vi "Measurement UI.vi"() -> ()   [LabVIEW 2021, in "Stepped Frequency Sweep_Class D Amplifier_UI.lvlib"]
uses:
  Stepped Frequency Sweep_Class D Amplifier_UI.lvlib
  shared/controls/sweep profile.ctl
  shared/controls/units - snr.ctl
  shared/controls/units - ratio.ctl
  Y axis data selection.ctl
  shared/controls/digital output level units.ctl
  shared/ui/controls/view.ctl
  UI State.ctl
  <vilib>/Utility/miscctls.llb/LVBoundsTypeDef.ctl
  <vilib>/Utility/miscctls.llb/LVPoint32TypeDef.ctl
  shared/ui/UI Helpers.lvlib
  shared/controls/audio controls.lvlib
panel:
  in  "view legend":T1
  out "Sweep graph":cluster{"frequency (Hz)":dbl[], "THD+N":dbl[]}[](graph)
  out "Time domain graph":waveform(dbl)(graph)
  out "Frequency domain graph":T2(graph)
  out "amplitude (Vrms)":dbl[](array[numeric])
  out "output power (W)":dbl[](array[numeric])
  out "SFDR (dBc)":dbl[](array[numeric])
  out "gain":dbl[](array[numeric])
  out "dynamic range (dB)":dbl[](array[numeric])
  out "THD":dbl[](array[numeric])
  out "THD+N":dbl[](array[numeric])
  out "SNR":dbl[](array[numeric])
  out "amplitude (dBFS)":dbl[](array[numeric])
  out "frequency (Hz)":dbl[](array[numeric])
  in  "Configuration tab":T3(tab)
  in  "enable dither":bool caption="Enable dither"
  in  "master clock channel list":string caption="Master Clock Channel"
  in  "digital channel list":string caption="Digital Audio Channel"
  in  "logic level":enum32{"3.3 V", "1.8 V", "1.2 V"}(ring) caption="Logic level"
  in  "master clock rate":dbl=12288000.0 caption="Master clock rate" format="%#_6pHz"
  out "Bit clock rate":dbl=3072000.0 format="%#_6pHz"
  in  "number of channels":u32=2 caption="Number of channels"
  in  "TDM":bool
  in  "RJ":bool
  in  "LJ":bool
  in  "I2S":bool
  in  "bit clock edge sync":enum32{"Rising", "Falling"}(ring)=enum."Falling" caption="Bit clock edge sync"
  in  "frame clock rate":dbl=48000.0 caption="Frame clock rate" format="%#_6pHz"
  in  "data justification":enum32{"Left Justified", "Right Justified"}(ring) caption="Data justification"
  in  "endianness":enum32{"MSB First", "LSB First"}(ring) caption="Endianness"
  in  "bit depth":u32=24 caption="Bit depth"
  in  "channel length":u32=32 caption="Channel length"
  in  "frame sync edge for channel 0":enum32{"Rising", "Falling"}(ring)=enum."Falling" caption="Frame sync edge for Channel 0"
  in  "output level":dbl=-1.0 caption="Output level" format="%#_3f"
  in  "output level units":T4
  in  "min settling cycles":u32 caption="Minimum settling cycles"
  in  "min settling time (s)":dbl=0.1 caption="Minimum settling time" format="%#_6ps"
  in  "sweep profile":T5=enum."Logarithmic" caption="Profile"
  in  "number of steps":u32=20000 caption="Number of steps"
  in  "sweep start frequency (Hz)":dbl=20.0 caption="Sweep start" format="%#_6pHz"
  in  "sweep stop frequency (Hz)":dbl=20000.0 caption="Sweep stop" format="%#_6pHz"
  in  "min measurement cycles":u32 caption="Minimum measurement cycles"
  in  "Acquisition channel":tag
  in  "acq sampling rate":dbl=51200.0 caption="Sample rate" format="%#.6pHz"
  in  "min measurement time (s)":dbl=0.1 caption="Minimum measurement time" format="%#_6ps"
  in  "lowpass filter":T6(ring) caption="Lowpass filter"
  in  "highpass filter":enum32{"DC", "AC"}(ring) caption="Highpass filter"
  in  "band start":dbl=20.0 caption="Band start" format="%#_6pHz"
  in  "band stop":dbl=20000.0 caption="Band stop" format="%#_6pHz"
  in  "weighting filter":T7(ring)=enum."A-weighting" caption="Weighting filter"
  in  "load impedance":dbl=4.0 caption="Load impedance" format="%#_6p Ohms"
  in  "output range (pk-pk)":dbl=15.0 caption="Output range" format="%.3p Vpk-pk"
  in  "gain units":T8 caption="Gain"
  in  "THD units":T8 caption="THD"
  in  "THD+N units":T8 caption="THD+N"
  in  "SNR units":T9 caption="SNR"
  in  "x-axis mapping":enum32{"linear", "logarithmic"}(ring) caption="X-axis mapping"
  in  "y-axis mapping":enum32{"linear", "logarithmic"}(ring) caption="Y-axis mapping"
  in  "y-axis data":T10 caption="Y-axis"
  in  "channel 0 offset":u32=1
  out "fft - data":dbl[](array[numeric])
  out "fft - df":dbl
  out "fft - f0":dbl
  out "wfm - data":dbl[](array[numeric])
  out "wfm - dt":dbl
  out "wfm - t0":dbl
  out "channel name":string
  in  "acq channel":string="PXI1Slot4/ai0"
  in  "signal phase":dbl caption="phase"
  # "hidden controls - used to sync with MeasLink"
  # "hidden indicators"
  # "Protocols"
  # "Audio Protocol"
  # "Clock Settings"
  # "Signal Level"
  # "Harware Resource"
  # "Sweep"
  # "Filters"
  # "Output"
  # "Acquisition"
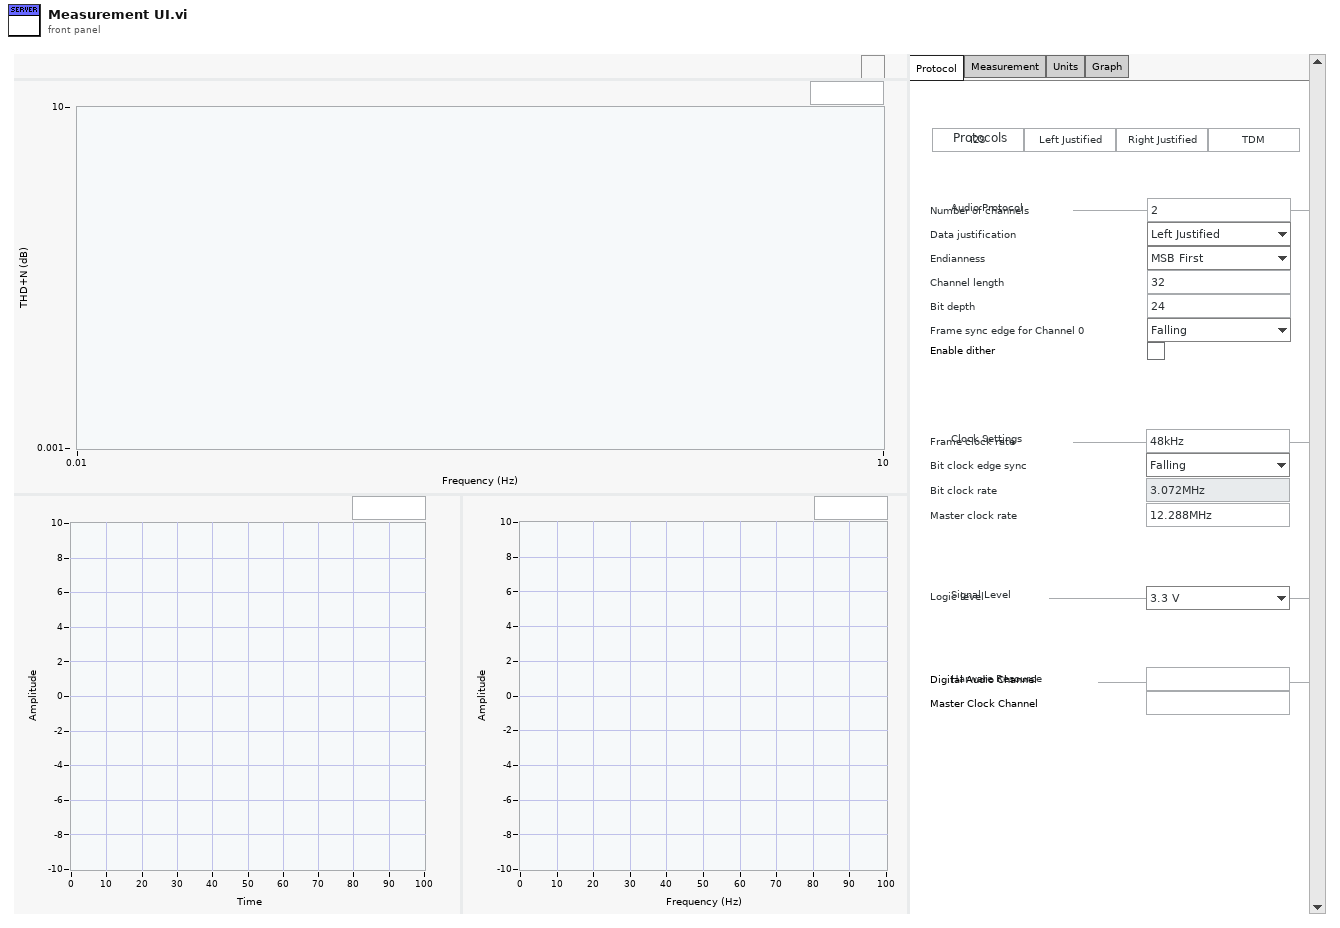
[diagram p1: front panel]
types:
  T1 = typedef "UI Helpers.lvlib/view.ctl" = bool
  T2 = cluster{"fft - f0":dbl, "fft - df":dbl, "fft - data":dbl[]}
  T3 = enum32{"Protocol", "Measurement", "Units", "Graph"}
  T4 = typedef "audio controls.lvlib/digital output level units.ctl" = enum32{"% FS", "dBFS"}
  T5 = typedef "audio controls.lvlib/sweep profile.ctl" = enum32{"Linear", "Logarithmic"}
  T6 = enum32{"No filter", "AES17 20kHz", "AES17 40kHz"}
  T7 = enum32{"Linear", "A-weighting", "B-weighting", "C-weighting"}
  T8 = typedef "audio controls.lvlib/units - ratio.ctl" = enum32{"dB", "%", "x/y"}
  T9 = typedef "audio controls.lvlib/units - snr.ctl" = enum32{"dB", "x/y"}
  T10 = typedef "Stepped Frequency Sweep_Class D Amplifier_UI.lvlib/Y axis data selection.ctl" = enum32{"THD+N", "THD", "Dynamic Range (dB)", "SFDR (dBc)", "SNR", "Gain", "Amplitude (dBFS)", "Amplitude (Vrms)", "Output Power (W)"}
  T11 = typedef "Stepped Frequency Sweep_Class D Amplifier_UI.lvlib/UI State.ctl" = cluster{"Graph Size":T12, "Legend Visible":bool, "Mouse Coords":T13}
  T12 = typedef "LVBoundsTypeDef.ctl" = cluster{"Width":u32, "Height":u32}
  T13 = typedef "LVPoint32TypeDef.ctl" = cluster{"Horizontal":i32, "Vertical":i32}
  T14 = cluster{"frequency (Hz)":dbl[], "amplitude (dBFS)":dbl[]}
  T15 = cluster{"frequency (Hz)":dbl[], "amplitude (Vrms)":dbl[]}
  T16 = cluster{"frequency (Hz)":dbl[], "output power (W)":dbl[]}
  T17 = cluster{"frequency (Hz)":dbl[], "dynamic range (dB)":dbl[]}
  T18 = cluster{"frequency (Hz)":dbl[], "SFDR (dBc)":dbl[]}
  T19 = cluster{"frequency (Hz)":dbl[], "SFDR (dBc)":dbl[]}[]
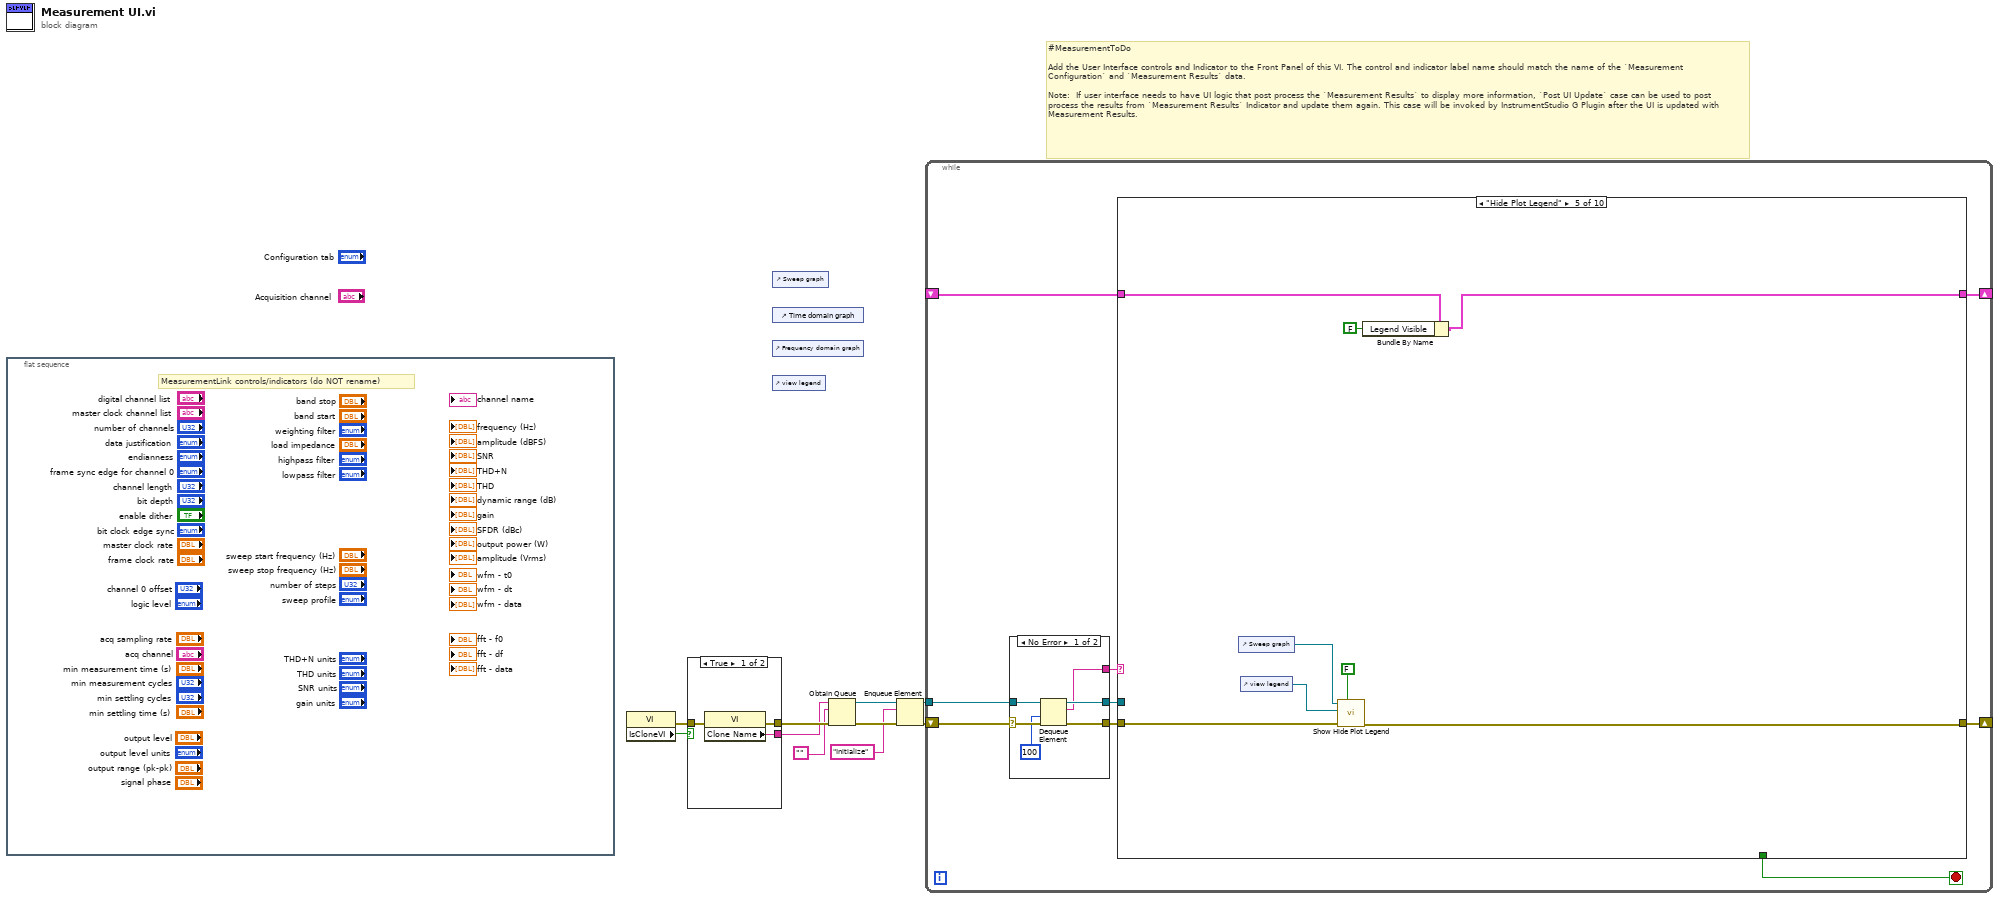
[diagram p0: block diagram]
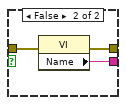
[diagram p2: hidden frame]
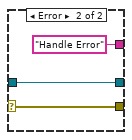
[diagram p3: hidden frame]
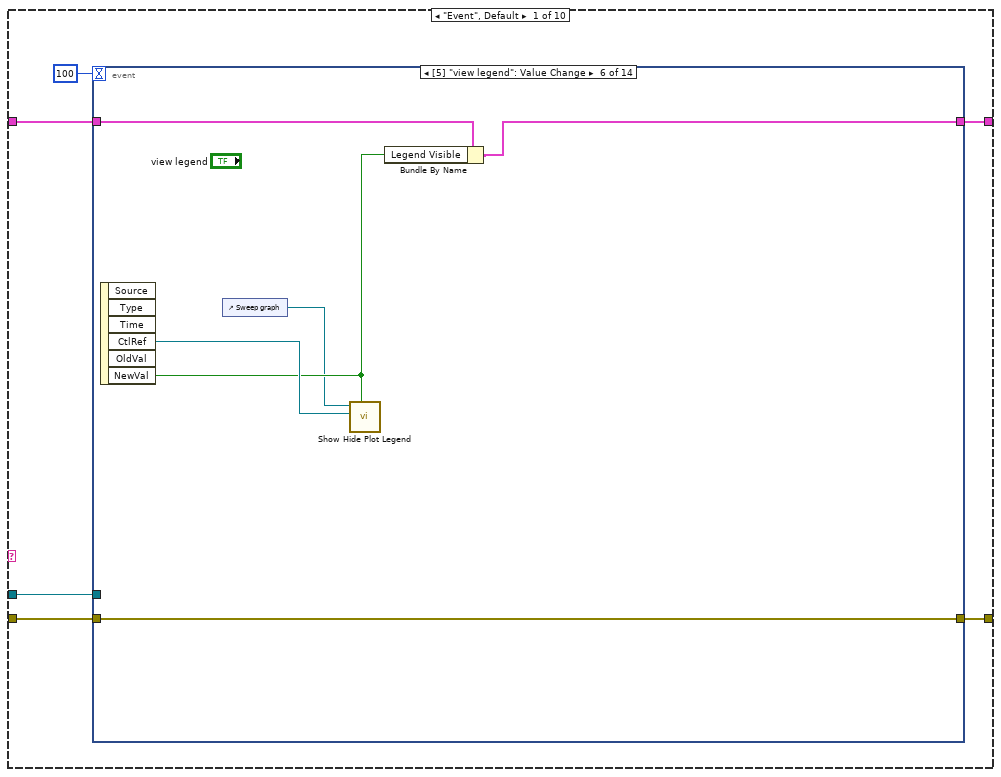
[diagram p4: hidden frame]
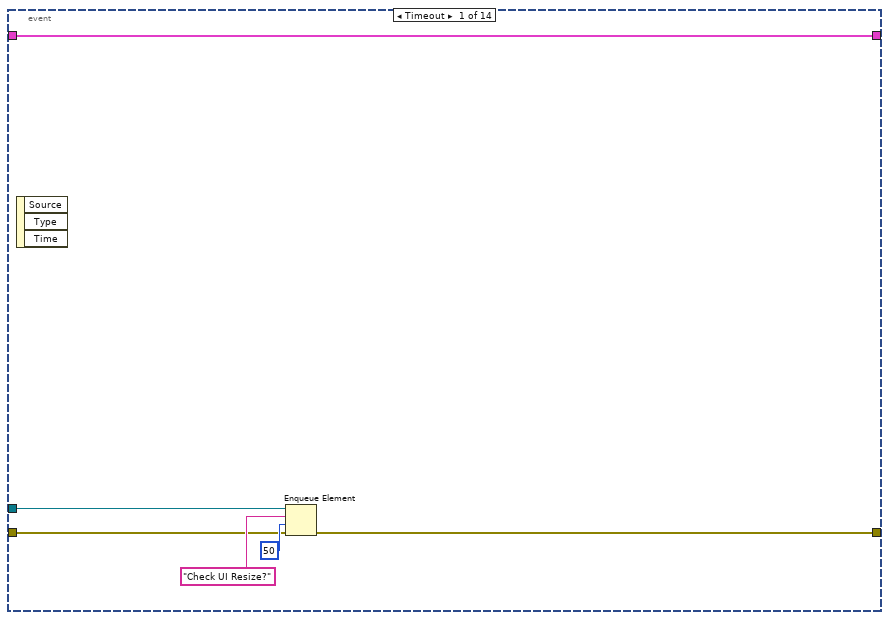
[diagram p5: hidden frame]
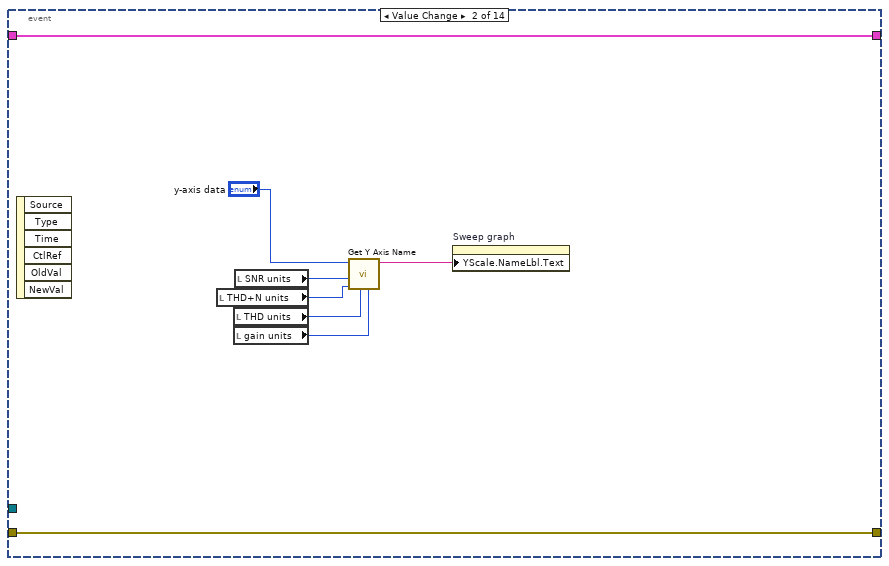
[diagram p6: hidden frame]
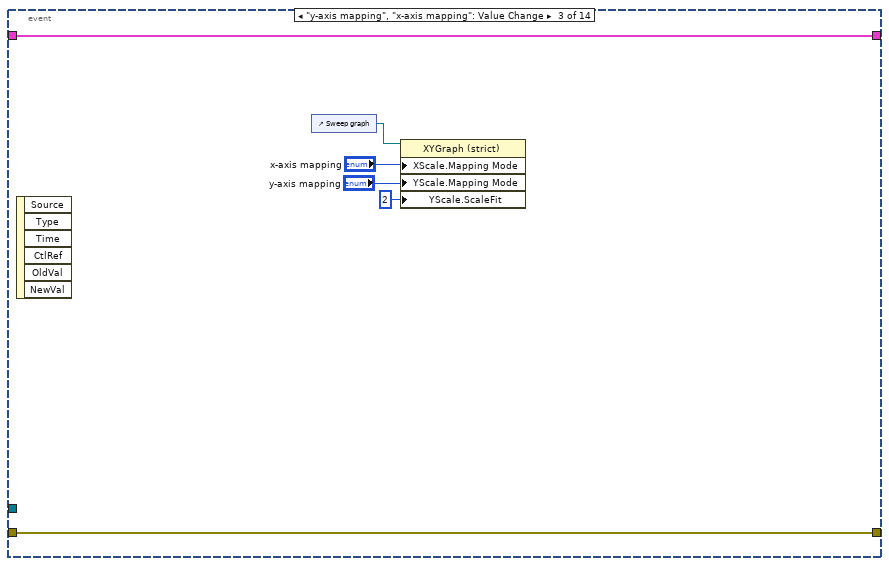
[diagram p7: hidden frame]
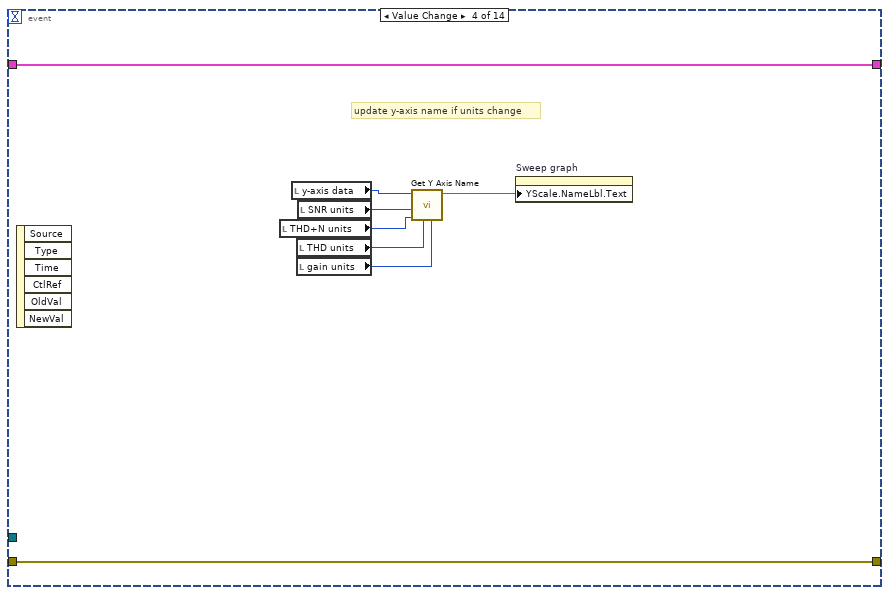
[diagram p8: hidden frame]
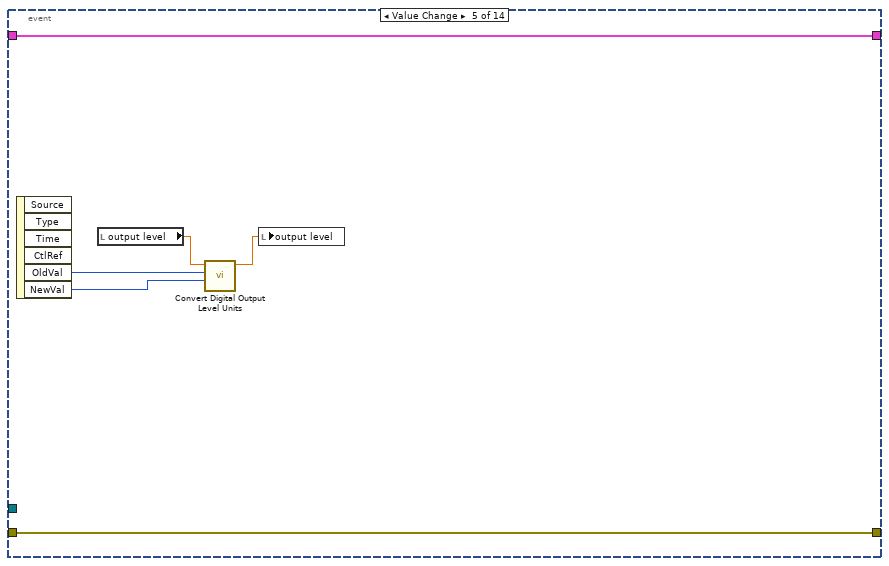
[diagram p9: hidden frame]
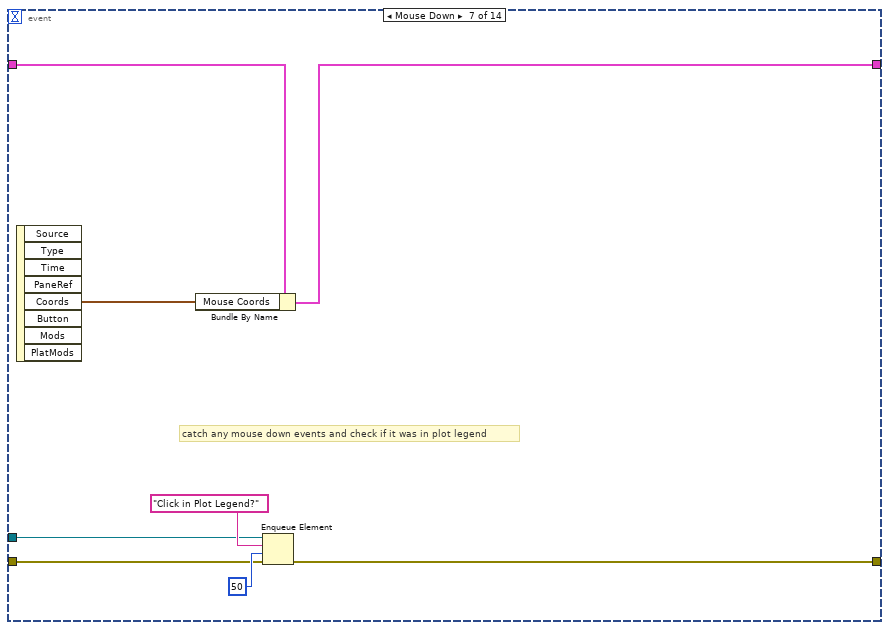
[diagram p10: hidden frame]
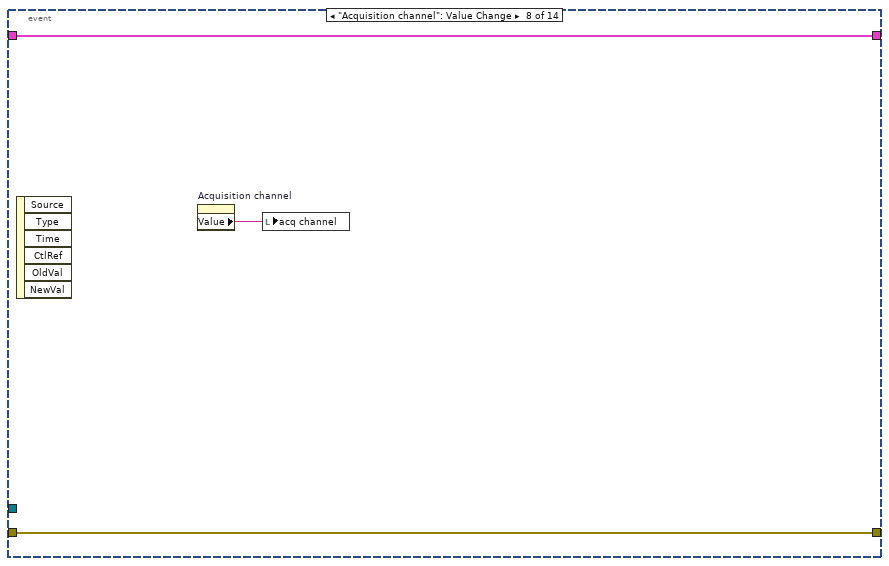
[diagram p11: hidden frame]
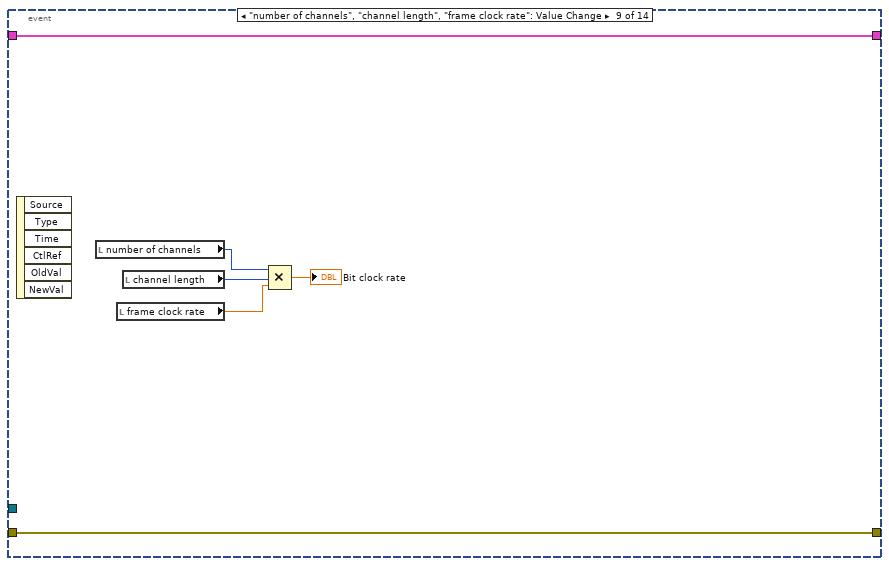
[diagram p12: hidden frame]
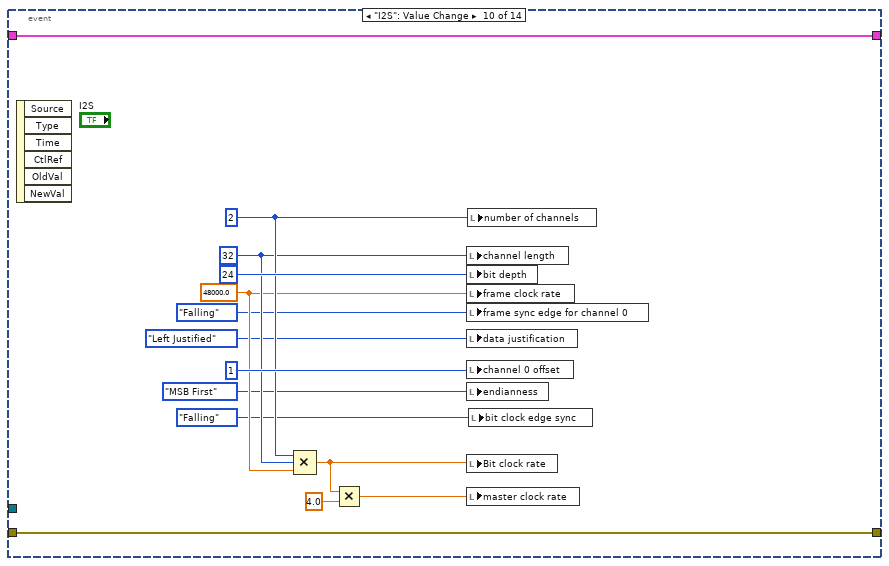
[diagram p13: hidden frame]
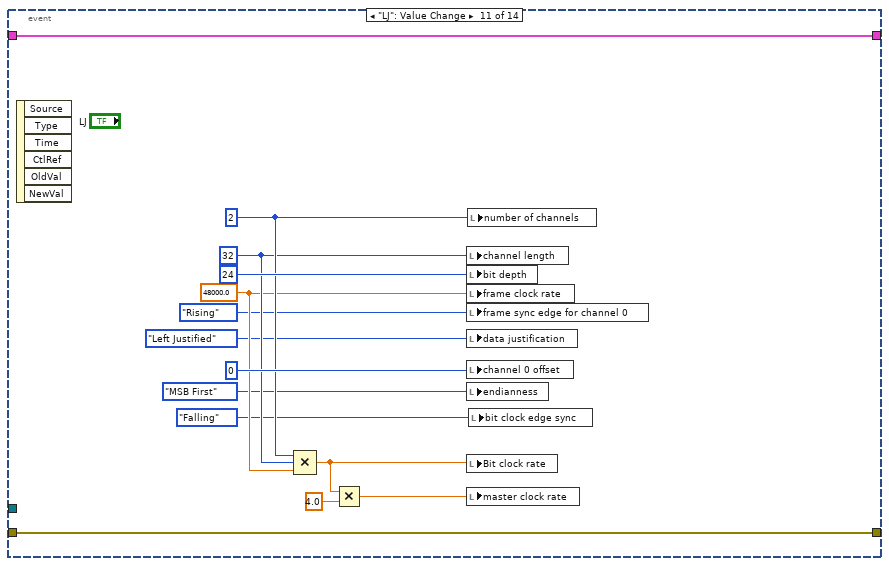
[diagram p14: hidden frame]
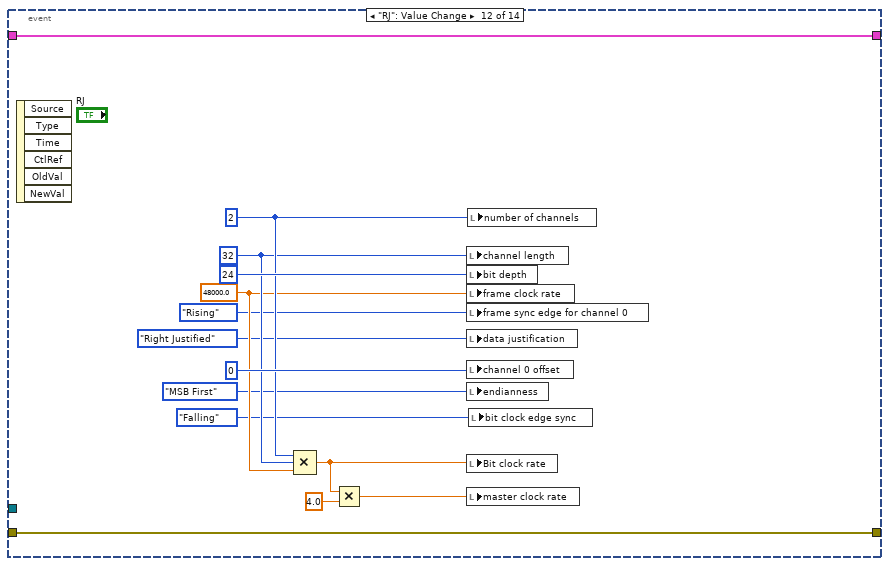
[diagram p15: hidden frame]
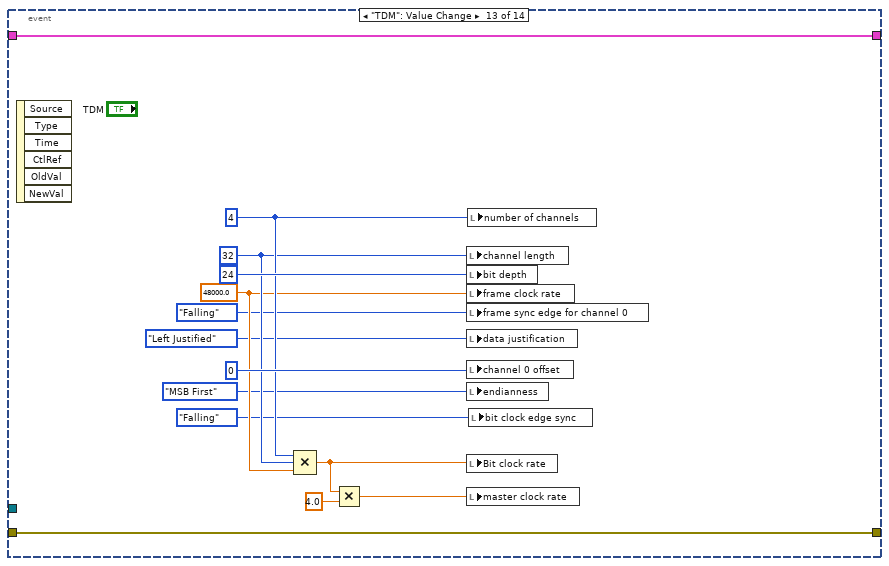
[diagram p16: hidden frame]
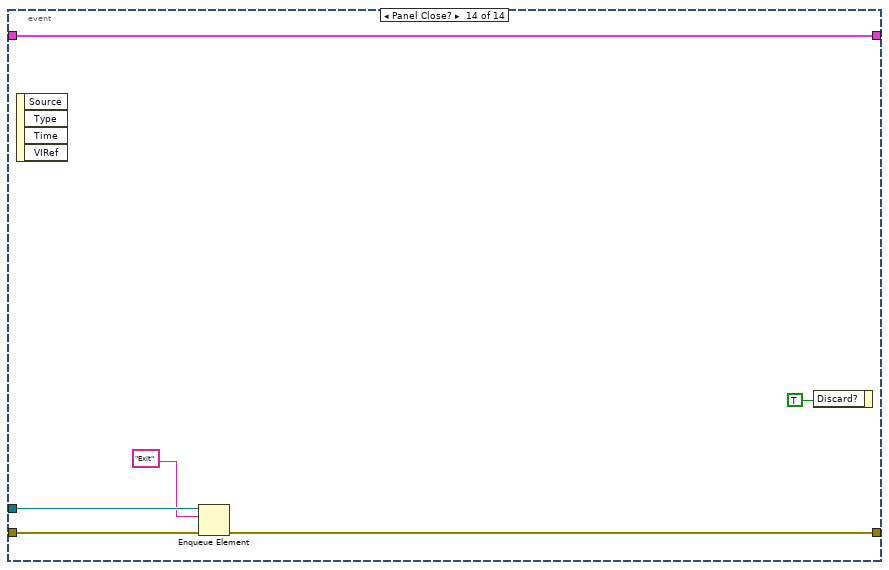
[diagram p17: hidden frame]
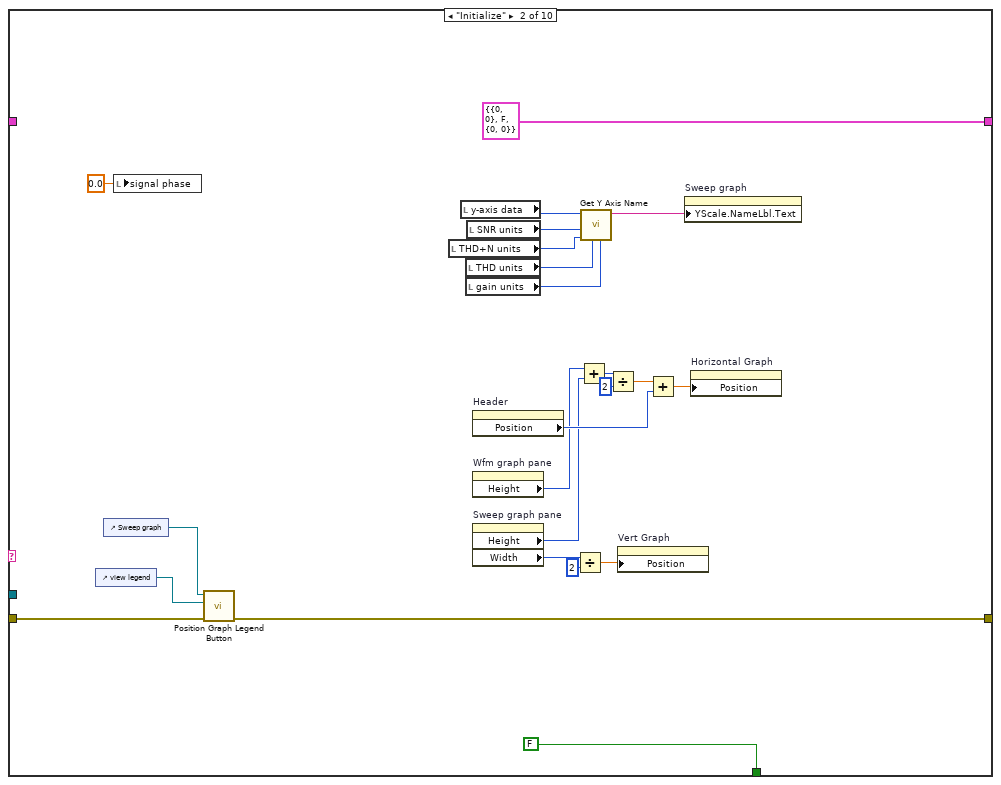
[diagram p18: hidden frame]
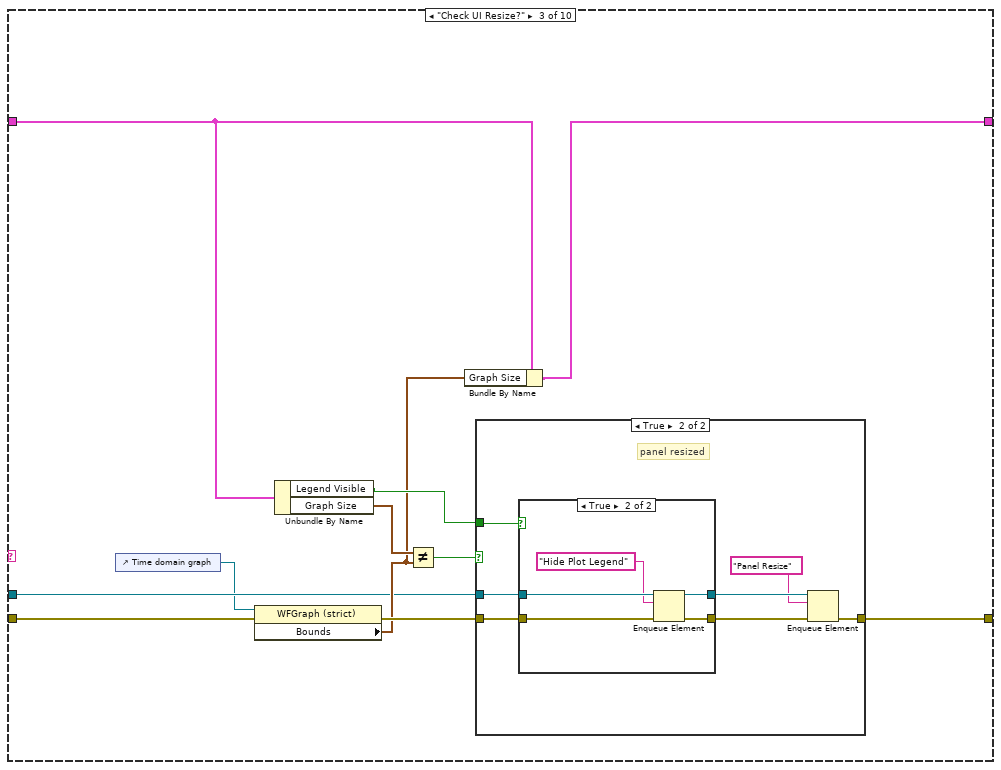
[diagram p19: hidden frame]
diagram:
  # "#MeasurementToDo  \n\nAdd the User Interface controls and Indicator to the Front Panel of this VI. The control and indicator label name should match the name of the `Measurement Configuration` and `Measurement Results` data.\n\nNote:  If user interface needs to have UI logic that post process the `Measurement Results` to display more information, `Post UI Update` case can be used to post process the results from `Measurement Results` Indicator and update them again. This case will be invoked by InstrumentStudio G Plugin after the UI is updated with Measurement Results."
  n1 = flat-sequence {
    frame #0 {
      # "MeasurementLink controls/indicators (do NOT rename)"
    }
  }
  n2 = property class="VI"() -> (error out=w1:errorcluster, "IsCloneVI"=w2:bool)  [unwired: 2 in, 1 out]
  n3 = case shown="True" w2 {
    tunnel: [w13 w16] -> w10
    tunnel: [w12 w15] -> w9
    tunnel: w1 -> [w11 w14]
    frame True {
      n4 = property class="VI"(error in=w11) -> (error out=w13:errorcluster, "Clone Name"=w12:string)  [unwired: 1 in, 1 out]
    }
    frame False {
      n5 = property class="VI"(error in=w14) -> (error out=w16:errorcluster, "Name"=w15:string)  [unwired: 1 in, 1 out]
    }
  }
  n6 = control-ref of="Sweep graph"() -> ()  [unwired: 1 out]
  n7 = control-ref of="Time domain graph"() -> ()  [unwired: 1 out]
  n8 = control-ref of="Frequency domain graph"() -> ()  [unwired: 1 out]
  n9 = control-ref of="view legend"() -> ()  [unwired: 1 out]
  n10 = Obtain Queue(name (unnamed)=w9, element data type="", error in (no error)=w10) -> (queue out=w6:refnum<queue>, error out=w8:errorcluster)  [unwired: 2 in, 1 out]
  n11 = Enqueue Element(queue=w6, element="Initialize", error in (no error)=w8) -> (queue out=w5:refnum<queue>, error out=w7:errorcluster)  [unwired: 1 in, 1 out]
  n12 = while {
    shift-right: [w20] -> _
    shift-left: w7 -> [w25]
    tunnel: w5 -> [w23]
    shift-right: [w18] -> _
    shift-left: _ -> [w17]
    stop <- w19 stop-if-true
    n13 = case shown="No Error" w25 {
      selector: w25 -> [w31 w34]
      tunnel: [w30 w34] -> w24
      tunnel: w23 -> [w29 w33]
      tunnel: [w28 w33] -> w22
      tunnel: [w27 "Handle Error"] -> w21
      frame No Error {
        n14 = Dequeue Element(queue=w29, timeout in ms (-1)=100, error in (no error)=w31) -> (queue out=w28:refnum<queue>, element=w27:string, error out=w30:errorcluster)  [unwired: 1 out]
      }
      frame Error {
      }
    }
    n15 = case shown="\"Hide Plot Legend\"" w21 {
      tunnel: w24 -> [w39 w174 w187 w211 w231 w239 w244 w277 w295 w297]
      tunnel: w22 -> [w37 _ w188 w212 _ _ w243 _ w293 _]
      tunnel: [w40 w173 w186 w210 w230 w238 w242 w277 w290 w297] -> w20
      tunnel: [_ FALSE _ _ _ _ _ _ TRUE _] -> w19
      tunnel: [w35 T11 {"Graph Size"={"Width"=0, "Height"=0}, "Legend Visible"=FALSE, "Mouse Coords"={"Horizontal"=0, "Vertical"=0}} ("UI State") w183 w209 w233 w240 w241 w276 w288 w296] -> w18
      tunnel: w17 -> [w36 _ w184 w209 w234 w240 w241 w276 w288 w296]
      frame "Event", Default {
        n16 = event shown="[5] \"view legend\": Value Change" {
          selector: _ -> [_ _ _ _ _ _ _ _ _ _ _ _ _ _]
          dyn-events: _ -> [_ _ _ _ _ _ _ _ _ _ _ _ _ _]
          timeout: 100 -> [_ _ _ _ _ _ _ _ _ _ _ _ _ _]
          tunnel: [w43 w47 w55 w61 w69 w80 w84 w89 w92 w98 w112 w126 w140 w157] -> w40
          tunnel: w39 -> [w44 w47 w55 w61 w69 w80 w86 w89 w92 w98 w112 w126 w140 w158]
          tunnel: w37 -> [w42 _ _ _ _ _ w85 _ _ _ _ _ _ w156]
          tunnel: w36 -> [w41 w48 w56 w62 w70 w77 w82 w90 w93 w99 w113 w127 w141 w154]
          tunnel: [w41 w48 w56 w62 w70 w76 w81 w90 w93 w99 w113 w127 w141 w154] -> w35
          event Timeout {
            n17 = event-data() -> ()  [unwired: 1 in, 3 out]
            n18 = Enqueue Element(queue=w42, element="Check UI Resize?", timeout in ms (-1)=50, error in (no error)=w44) -> (error out=w43:errorcluster)  [unwired: 2 out]
          }
          event Value Change {
            n19 = event-data() -> ()  [unwired: 1 in, 6 out]
            n20 = local read "THD+N units"() -> (w52:T8)
            n21 = local read "THD units"() -> (w51:T8)
            n22 = local read "gain units"() -> (w50:T8)
            n23 = local read "SNR units"() -> (w53:T9)
            n24 = call "Get Y Axis Name.vi"("gain units"=w50, "THD units"=w51, "THD+N units"=w52, "SNR units"=w53, "y-axis data"="y-axis data") -> ("units"=w49:string)  [unwired: 6 in]
            n25 = property on="Sweep graph" class="XYGraph (strict)"("YScale.NameLbl.Text"=w49) -> ()  [unwired: 2 in, 2 out]
          }
          event "y-axis mapping", "x-axis mapping": Value Change {
            n26 = event-data() -> ()  [unwired: 1 in, 6 out]
            n27 = control-ref of="Sweep graph"() -> (w58:refnum<vi>)
            n28 = property on="Property Node" class="XYGraph (strict)"(reference=w58, "XScale.Mapping Mode"="x-axis mapping", "YScale.Mapping Mode"="y-axis mapping", "YScale.ScaleFit"=u8 2 ("Y Scale.Scale Fit")) -> ()  [unwired: 1 in, 2 out]
          }
          event Value Change {
            # "update y-axis name if units change"
            n29 = event-data() -> ()  [unwired: 1 in, 6 out]
            n30 = local read "THD+N units"() -> (w67:T8)
            n31 = local read "y-axis data"() -> (w63:T10)
            n32 = local read "THD units"() -> (w66:T8)
            n33 = local read "gain units"() -> (w65:T8)
            n34 = local read "SNR units"() -> (w68:T9)
            n35 = call "Get Y Axis Name.vi"("gain units"=w65, "THD units"=w66, "THD+N units"=w67, "SNR units"=w68, "y-axis data"=w63) -> ("units"=w64:string)  [unwired: 6 in]
            n36 = property on="Sweep graph" class="XYGraph (strict)"("YScale.NameLbl.Text"=w64) -> ()  [unwired: 2 in, 2 out]
          }
          event Value Change {
            n37 = event-data() -> ("OldVal"=w74:T4, "NewVal"=w73:T4)  [unwired: 1 in, 4 out]
            n38 = local read "output level"() -> (w71:dbl)
            n39 = call "Convert Digital Output Level Units.vi"("new output level units"=w73, "previous output level units"=w74, "previous output level"=w71) -> ("new output level"=w72:dbl)  [unwired: 8 in]
            n40 = local write "output level"(w72) -> ()
          }
          event Value Change {
            n41 = event-data() -> ("CtlRef"=w79:refnum<vi>, "NewVal"=w78:T1)  [unwired: 1 in, 4 out]
            n42 = control-ref of="Sweep graph"() -> (w75:refnum<vi>)
            n43 = call "Show Hide Plot Legend.vi"("show"=w78, "view reference"=w79, "graph reference"=w75) -> ()  [unwired: 8 in, 1 out]
            n44 = Bundle By Name(cluster=w77, "Legend Visible"=w78) -> (w76:T11)
          }
          event Mouse Down {
            # "catch any mouse down events and check if it was in plot legend"
            n45 = event-data() -> ("Coords"=w83:T13)  [unwired: 1 in, 7 out]
            n46 = Bundle By Name(cluster=w82, "Mouse Coords"=w83) -> (w81:T11)
            n47 = Enqueue Element(queue=w85, element="Click in Plot Legend?", timeout in ms (-1)=50, error in (no error)=w86) -> (error out=w84:errorcluster)  [unwired: 2 out]
          }
          event "Acquisition channel": Value Change {
            n48 = event-data() -> ()  [unwired: 1 in, 6 out]
            n49 = property on="Acquisition channel" class="DAQmxName"() -> ("Value"=w91:string)  [unwired: 2 in, 2 out]
            n50 = local write "acq channel"(w91) -> ()
          }
          event "number of channels", "channel length", "frame clock rate": Value Change {
            n51 = event-data() -> ()  [unwired: 1 in, 6 out]
            n52 = local read "number of channels"() -> (w97:u32)
            n53 = local read "frame clock rate"() -> (w95:dbl)
            n54 = local read "channel length"() -> (w96:u32)
            n55 = Compound Arithmetic op=MULTIPLY(w97, w96, w95) -> (→"Bit clock rate":dbl)
          }
          event "I2S": Value Change {
            w107 = 48000.0 ("Frame Clock Rate")
            w108 = u32 32 ("Channel Length")
            w109 = u32 2 ("Number of Channels")
            n56 = event-data() -> ()  [unwired: 1 in, 6 out]
            n57 = Compound Arithmetic op=MULTIPLY(w109, w108, w107) -> (w106:dbl)
            n58 = Multiply(x=w106, y=4.0) -> (x*y=w105:dbl)
            n59 = local write "channel length"(w108) -> ()
            n60 = local write "bit depth"(u32 24 ("Bit Depth")) -> ()
            n61 = local write "frame clock rate"(w107) -> ()
            n62 = local write "frame sync edge for channel 0"(enum32{"Rising", "Falling"}."Falling" ("bit clock edge sync")) -> ()
            n63 = local write "data justification"(enum32{"Left Justified", "Right Justified"}."Left Justified" ("data justification")) -> ()
            n64 = local write "channel 0 offset"(u32 1 ("Channel 0 Offset")) -> ()
            n65 = local write "endianness"(enum32{"MSB First", "LSB First"}."MSB First" ("endianness")) -> ()
            n66 = local write "Bit clock rate"(w106) -> ()
            n67 = local write "master clock rate"(w105) -> ()
            n68 = local write "number of channels"(w109) -> ()
            n69 = local write "bit clock edge sync"(enum32{"Rising", "Falling"}."Falling" ("frame sync edge for channel 0")) -> ()
          }
          event "LJ": Value Change {
            w121 = 48000.0 ("Frame Clock Rate")
            w122 = u32 32 ("Channel Length")
            w123 = u32 2 ("Number of Channels")
            n70 = event-data() -> ()  [unwired: 1 in, 6 out]
            n71 = Compound Arithmetic op=MULTIPLY(w123, w122, w121) -> (w120:dbl)
            n72 = Multiply(x=w120, y=4.0) -> (x*y=w119:dbl)
            n73 = local write "channel length"(w122) -> ()
            n74 = local write "bit depth"(u32 24 ("Bit Depth")) -> ()
            n75 = local write "frame clock rate"(w121) -> ()
            n76 = local write "frame sync edge for channel 0"(enum32{"Rising", "Falling"}."Rising" ("bit clock edge sync")) -> ()
            n77 = local write "data justification"(enum32{"Left Justified", "Right Justified"}."Left Justified" ("data justification")) -> ()
            n78 = local write "channel 0 offset"(u32 0 ("Channel 0 Offset")) -> ()
            n79 = local write "endianness"(enum32{"MSB First", "LSB First"}."MSB First" ("endianness")) -> ()
            n80 = local write "Bit clock rate"(w120) -> ()
            n81 = local write "master clock rate"(w119) -> ()
            n82 = local write "number of channels"(w123) -> ()
            n83 = local write "bit clock edge sync"(enum32{"Rising", "Falling"}."Falling" ("frame sync edge for channel 0")) -> ()
          }
          event "RJ": Value Change {
            w135 = 48000.0 ("Frame Clock Rate")
            w136 = u32 32 ("Channel Length")
            w137 = u32 2 ("Number of Channels")
            n84 = event-data() -> ()  [unwired: 1 in, 6 out]
            n85 = Compound Arithmetic op=MULTIPLY(w137, w136, w135) -> (w134:dbl)
            n86 = Multiply(x=w134, y=4.0) -> (x*y=w133:dbl)
            n87 = local write "channel length"(w136) -> ()
            n88 = local write "bit depth"(u32 24 ("Bit Depth")) -> ()
            n89 = local write "frame clock rate"(w135) -> ()
            n90 = local write "frame sync edge for channel 0"(enum32{"Rising", "Falling"}."Rising" ("bit clock edge sync")) -> ()
            n91 = local write "data justification"(enum32{"Left Justified", "Right Justified"}."Right Justified" ("data justification")) -> ()
            n92 = local write "channel 0 offset"(u32 0 ("Channel 0 Offset")) -> ()
            n93 = local write "endianness"(enum32{"MSB First", "LSB First"}."MSB First" ("endianness")) -> ()
            n94 = local write "Bit clock rate"(w134) -> ()
            n95 = local write "master clock rate"(w133) -> ()
            n96 = local write "number of channels"(w137) -> ()
            n97 = local write "bit clock edge sync"(enum32{"Rising", "Falling"}."Falling" ("frame sync edge for channel 0")) -> ()
          }
          event "TDM": Value Change {
            w149 = 48000.0 ("Frame Clock Rate")
            w150 = u32 32 ("Channel Length")
            w151 = u32 4 ("Number of Channels")
            n98 = event-data() -> ()  [unwired: 1 in, 6 out]
            n99 = Compound Arithmetic op=MULTIPLY(w151, w150, w149) -> (w148:dbl)
            n100 = Multiply(x=w148, y=4.0) -> (x*y=w147:dbl)
            n101 = local write "channel length"(w150) -> ()
            n102 = local write "bit depth"(u32 24 ("Bit Depth")) -> ()
            n103 = local write "frame clock rate"(w149) -> ()
            n104 = local write "frame sync edge for channel 0"(enum32{"Rising", "Falling"}."Falling" ("bit clock edge sync")) -> ()
            n105 = local write "data justification"(enum32{"Left Justified", "Right Justified"}."Left Justified" ("data justification")) -> ()
            n106 = local write "channel 0 offset"(u32 0 ("Channel 0 Offset")) -> ()
            n107 = local write "endianness"(enum32{"MSB First", "LSB First"}."MSB First" ("endianness")) -> ()
            n108 = local write "Bit clock rate"(w148) -> ()
            n109 = local write "master clock rate"(w147) -> ()
            n110 = local write "number of channels"(w151) -> ()
            n111 = local write "bit clock edge sync"(enum32{"Rising", "Falling"}."Falling" ("frame sync edge for channel 0")) -> ()
          }
          event Panel Close? {
            n112 = event-data() -> ()  [unwired: 1 in, 4 out]
            n113 = Enqueue Element(queue=w156, element="Exit", error in (no error)=w158) -> (error out=w157:errorcluster)  [unwired: 1 in, 2 out]
            n114 = event-data("Discard?"=TRUE) -> ()  [unwired: 1 in, 1 out]
          }
        }
      }
      frame "Initialize" {
        n115 = control-ref of="view legend"() -> (w172:refnum<vi>)
        n116 = control-ref of="Sweep graph"() -> (w171:refnum<vi>)
        n117 = local write "signal phase"(0.0 ("signal phase")) -> ()
        n118 = call "Position Graph Legend Button.vi"("error in (no error)"=w174, "view legend"=w172, "graph"=w171) -> ("error out"=w173:errorcluster)  [unwired: 8 in]
        n119 = local read "THD+N units"() -> (w177:T8)
        n120 = local read "y-axis data"() -> (w175:T10)
        n121 = local read "THD units"() -> (w178:T8)
        n122 = local read "gain units"() -> (w179:T8)
        n123 = local read "SNR units"() -> (w176:T9)
        n124 = property on="Header" class="Splitter"() -> ("Position"=w164:i32)  [unwired: 2 in, 2 out]
        n125 = property on="Wfm graph pane" class="Pane"() -> ("Height"=w163:u32)  [unwired: 2 in, 2 out]
        n126 = property on="Sweep graph pane" class="Pane"() -> ("Height"=w162:u32, "Width"=w166:u32)  [unwired: 2 in, 2 out]
        n127 = Divide(x=w166, y=2) -> (x/y=w165:dbl)
        n128 = Add(x=w163, y=w162) -> (x+y=w161:u32)
        n129 = call "Get Y Axis Name.vi"("gain units"=w179, "THD units"=w178, "THD+N units"=w177, "SNR units"=w176, "y-axis data"=w175) -> ("units"=w180:string)  [unwired: 6 in]
        n130 = Divide(x=w161, y=2) -> (x/y=w169:dbl)
        n131 = property on="Vert Graph" class="Splitter"("Position"=w165) -> ()  [unwired: 2 in, 2 out]
        n132 = Add(x=w169, y=w164) -> (x+y=w168:dbl)
        n133 = property on="Sweep graph" class="XYGraph (strict)"("YScale.NameLbl.Text"=w180) -> ()  [unwired: 2 in, 2 out]
        n134 = property on="Horizontal Graph" class="Splitter"("Position"=w168) -> ()  [unwired: 2 in, 2 out]
      }
      frame "Check UI Resize?" {
        n135 = control-ref of="Time domain graph"() -> (w185:refnum<vi>)
        n136 = property on="Property Node" class="WFGraph (strict)"(reference=w185, error in=w187) -> (error out=w193:errorcluster, "Bounds"=w189:T12)  [unwired: 1 out]
        n137 = Unbundle By Name(w184) -> ("Legend Visible"=w191:bool, "Graph Size"=w190:T12)
        n138 = Not Equal?(x=w190, y=w189) -> (x != y?=w192:bool)
        n139 = Bundle By Name(cluster=w184, "Graph Size"=w189) -> (w183:T11)
        n140 = case shown="True" w192 {
          tunnel: w193 -> [w194 w201]
          tunnel: [w194 w196] -> w186
          tunnel: w191 -> [_ w199]
          tunnel: w188 -> [_ w200]
          frame False {
            # "no resize"
          }
          frame True {
            # "panel resized"
            n141 = case shown="True" w199 {
              tunnel: w201 -> [w203 w208]
              tunnel: [w203 w207] -> w198
              tunnel: w200 -> [w202 w206]
              tunnel: [w202 w204] -> w197
              frame False {
              }
              frame True {
                n142 = Enqueue Element(queue=w206, element="Hide Plot Legend", error in (no error)=w208) -> (queue out=w204:refnum<queue>, error out=w207:errorcluster)  [unwired: 1 in, 1 out]
              }
            }
            n143 = Enqueue Element(queue=w197, element="Panel Resize", error in (no error)=w198) -> (error out=w196:errorcluster)  [unwired: 1 in, 2 out]
          }
        }
      }
      frame "Click in Plot Legend?" {
        n144 = Unbundle By Name(w209) -> ("Legend Visible"=w213:bool, "Mouse Coords"=w214:T13)
        n145 = case shown="True" w213 {
          tunnel: w214 -> [_ w221]
          tunnel: w212 -> [_ w218]
          tunnel: w211 -> [w215 w222]
          tunnel: [w215 w217] -> w210
          frame False {
            # "legend not visible; do nothing"
          }
          frame True {
            # "check if mouse down in legend"
            n146 = control-ref of="Sweep graph"() -> (w216:refnum<vi>)
            n147 = call "Check if Click in Graph Legend.vi"("error in (no error)"=w222, "Mouse Coords"=w221, "WaveformGraph"=w216) -> ("error out"=w219:errorcluster, "click in legend?"=w220:bool)  [unwired: 7 in]
            n148 = case shown="True" w220 {
              tunnel: w219 -> [w226 w227]
              tunnel: w218 -> [w225 _]
              tunnel: [w224 w227] -> w217
              frame False {
                n149 = Enqueue Element(queue=w225, element="Hide Plot Legend", error in (no error)=w226) -> (error out=w224:errorcluster)  [unwired: 1 in, 2 out]
              }
              frame True {
                # "inside legend; do nothing"
              }
            }
          }
        }
      }
      frame "Hide Plot Legend" {
        n150 = control-ref of="Sweep graph"() -> (w228:refnum<vi>)
        n151 = control-ref of="view legend"() -> (w229:refnum<vi>)
        n152 = call "Show Hide Plot Legend.vi"("show"=FALSE, "error in (no error)"=w231, "view reference"=w229, "graph reference"=w228) -> ("error out"=w230:errorcluster)  [unwired: 7 in]
        n153 = Bundle By Name(cluster=w234, "Legend Visible"=FALSE ("legend visible")) -> (w233:T11)
      }
      frame "Panel Resize" {
        n154 = control-ref of="Sweep graph"() -> (w237:refnum<vi>)
        n155 = control-ref of="view legend"() -> (w236:refnum<vi>)
        n156 = call "Position Graph Legend Button.vi"("error in (no error)"=w239, "view legend"=w236, "graph"=w237) -> ("error out"=w238:errorcluster)  [unwired: 8 in]
      }
      frame "Post UI Update" {
        # "Initialize the DAQmx channel control"
        # "This case will be triggered, after framework updates the User interface with result values."
        n157 = for {
          tunnel: w243 -> [w249]
          shift-right: [w248] -> w242
          shift-left: w244 -> [w250]
          tunnel: string[] ["Update Graphs"] -> [w247] mode=indexing
          n158 = Enqueue Element(queue=w249, element=w247, timeout in ms (-1)=50, error in (no error)=w250) -> (error out=w248:errorcluster)  [unwired: 2 out]
        }
        n159 = local read "acq channel"() -> (w246:string)
        n160 = property on="Acquisition channel" class="DAQmxName"("Value"=w246) -> ()  [unwired: 2 in, 2 out]
      }
      frame "Update Graphs" {
        n161 = control-ref of="Sweep graph"() -> (w272:refnum<vi>)
        n162 = for {
          tunnel: string[] ["THD+N", "THD", "SNR", "Gain", "Amplitude (dBFS)", "Amplitude (Vrms)", "Output Power", "Dynamic Range", "SFDR"] -> [w286] mode=indexing
          tunnel: w272 -> [w285]
          i -> [w287]
          n163 = property on="Property Node" class="XYGraph (strict)"(reference=w285, "Active Plot"=w287, "Plot.Plot Name"=w286) -> ()  [unwired: 1 in, 2 out]
        }
        n164 = property class="XYGraph (strict)"(reference=w272, "LegNumRows"=u32 9 ("Legend:Number of Rows"), "LegScrollVis"=FALSE ("Legend:Scrollbar Visible")) -> ()  [unwired: 1 in, 2 out]
        n165 = local read "wfm - data"() -> (w283:dbl[])
        n166 = local read "fft - data"() -> (w280:dbl[])
        n167 = local read "wfm - dt"() -> (w282:dbl)
        n168 = local read "fft - df"() -> (w279:dbl)
        n169 = local read "fft - f0"() -> (w278:dbl)
        n170 = local read "dynamic range (dB)"() -> (w261:dbl[])
        n171 = local read "output power (W)"() -> (w262:dbl[])
        n172 = local read "amplitude (Vrms)"() -> (w263:dbl[])
        n173 = local read "amplitude (dBFS)"() -> (w264:dbl[])
        n174 = Bundle By Name("dt"=w282, "Y"=w283) -> (→"Time domain graph":waveform(dbl))  [unwired: 1 in]
        n175 = Bundle("fft - f0"=w278, "fft - df"=w279, "fft - data"=w280) -> (→"Frequency domain graph":T2)  [unwired: 1 in]
        n176 = local read "frequency (Hz)"() -> (w268:dbl[])
        n177 = local read "SFDR (dBc)"() -> (w260:dbl[])
        n178 = local read "THD+N"() -> (w271:dbl[])
        n179 = local read "THD"() -> (w267:dbl[])
        n180 = local read "gain"() -> (w265:dbl[])
        n181 = local read "SNR"() -> (w266:dbl[])
        n182 = Bundle("frequency (Hz)"=w268, "THD+N"=w271) -> (w270:cluster{"frequency (Hz)":dbl[], "THD+N":dbl[]})  [unwired: 1 in]
        n183 = Bundle("frequency (Hz)"=w268, "THD"=w267) -> (w259:cluster{"frequency (Hz)":dbl[], "THD":dbl[]})  [unwired: 1 in]
        n184 = Bundle("frequency (Hz)"=w268, "SNR"=w266) -> (w258:cluster{"frequency (Hz)":dbl[], "SNR":dbl[]})  [unwired: 1 in]
        n185 = Bundle("frequency (Hz)"=w268, "gain"=w265) -> (w257:cluster{"frequency (Hz)":dbl[], "gain":dbl[]})  [unwired: 1 in]
        n186 = Bundle("frequency (Hz)"=w268, "amplitude (dBFS)"=w264) -> (w256:T14)  [unwired: 1 in]
        n187 = Bundle("frequency (Hz)"=w268, "amplitude (Vrms)"=w263) -> (w255:T15)  [unwired: 1 in]
        n188 = Bundle("frequency (Hz)"=w268, "output power (W)"=w262) -> (w254:T16)  [unwired: 1 in]
        n189 = Bundle("frequency (Hz)"=w268, "dynamic range (dB)"=w261) -> (w253:T17)  [unwired: 1 in]
        n190 = Bundle("frequency (Hz)"=w268, "SFDR (dBc)"=w260) -> (w252:T18)  [unwired: 1 in]
        n191 = Build Array(w270, w259, w258, w257, w256, w255, w254, w253, w252) -> (→"Sweep graph":T19)
      }
      frame "Exit" {
        # "This case is triggered to close the User Interface from framework"
        n192 = Flush Queue(queue=w293, error in (no error)=w295) -> (queue out=w292:refnum<queue>, error out=w291:errorcluster)  [unwired: 1 out]
        n193 = Release Queue(queue=w292, force destroy? (F)=TRUE, error in (no error)=w291) -> (error out=w290:errorcluster)  [unwired: 2 out]
      }
      frame "Handle Error" {
      }
    }
  }
